vi "ECU Event Page.vi"(8 "error in (no error)":errorcluster, 11 "Node Ptr":T1 format="%.0x") -> (0 "error out":errorcluster)   [LabVIEW 2011, in "Engine Sim System Explorer.lvlib"]
uses:
  Engine Sim System Explorer.lvlib
  <vilib>/NI Veristand/Custom Device API/Custom Device Item Ref.ctl
  Shared/Engine Simulation Global.vi
  <vilib>/NI Veristand/Custom Device API/Get Item Property (Boolean).vi
  <vilib>/NI Veristand/Custom Device API/Get Item Property (Double).vi
  <vilib>/NI Veristand/Custom Device API/Set Item Property (Boolean).vi
  <vilib>/NI Veristand/Custom Device API/Set Item Property (Double).vi
  <vilib>/NI Veristand/Custom Device API/Custom Device API.lvlib
  Engine Simulation Shared.lvlib
panel:
  in  "ParentRate":bool
  in  "FPGA Event Loop Rate (Hz)":dbl format="%#_p"
  in  "SHDocVw.IWebBrowser2":refnum<k7>(container)
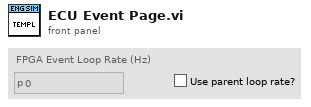
[diagram p1: front panel]
types:
  T1 = typedef "Custom Device API.lvlib/Custom Device Item Ref.ctl" = u64
  T2 = enum8{"Enabled", "Disabled", "Disabled and Grayed Out"}
  T3 = typedef "Custom Device API.lvlib/Custom Device Commands.ctl" = enum16{"Default", "Item renamed", "Shutdown", "Dynamic button pressed"}
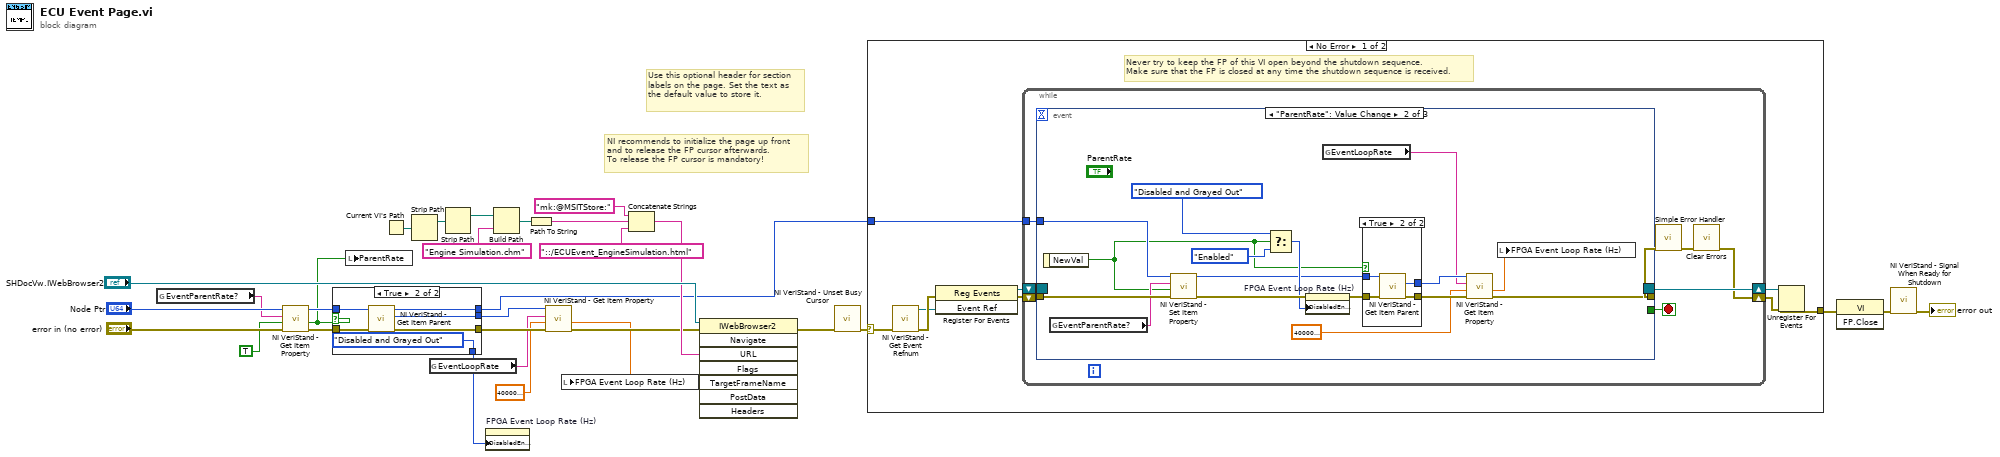
[diagram p0: block diagram]
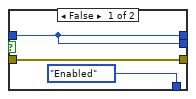
[diagram p2: hidden frame]
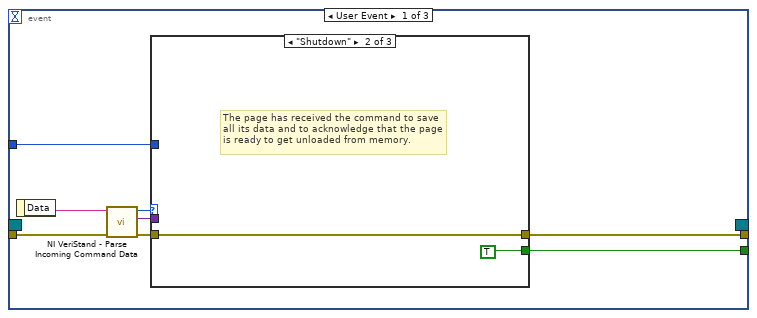
[diagram p3: hidden frame]
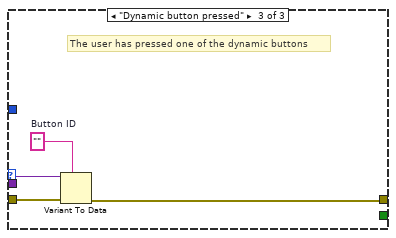
[diagram p5: hidden frame]
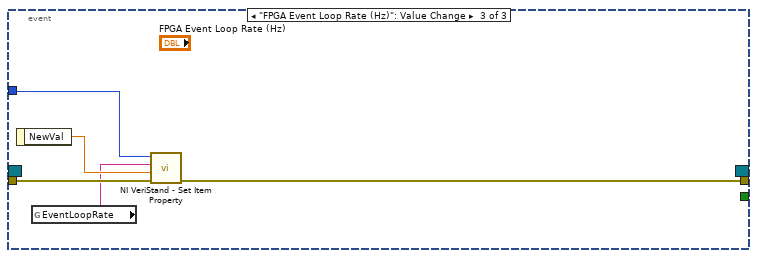
[diagram p7: hidden frame]
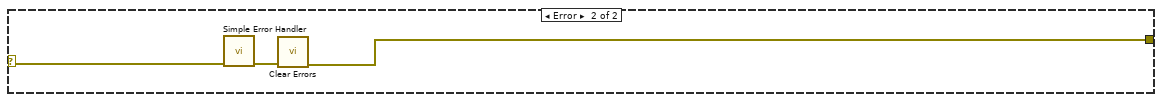
[diagram p8: hidden frame]
diagram:
  # "Use this optional header for section labels on the page. Set the text as the default value to store it."
  # "NI recommends to initialize the page up front\nand to release the FP cursor afterwards.\nTo release the FP cursor is mandatory!"
  n1 = global read "Engine Simulation Global.vi" "EventParentRate?"() -> (w13:string)
  n2 = call-poly <vilib>:"NI VeriStand - Get Item Property.vi"("error in (no error)"="error in (no error)", "Default Value"=TRUE, "Property Name"=w13, "Item Ref in"="Node Ptr") -> ("error out"=w10:errorcluster, "Value"=w9:bool, "Item Ref out"=w11:T1)  [unwired: 4 in, 1 out]
  n3 = case shown="True" w9 {
    tunnel: w11 -> [w32 w39]
    tunnel: w10 -> [w33 w38]
    tunnel: [w33 w37] -> w8
    tunnel: [w32 w36] -> w5
    tunnel: [w32 w35] -> w4
    tunnel: [T2."Enabled" ("Disabled") T2."Disabled and Grayed Out" ("Disabled")] -> w1
    frame False {
    }
    frame True {
      n4 = call <vilib>:"NI VeriStand - Get Item Parent.vi"("error in (no error)"=w38, "Item Ref in"=w39) -> ("error out"=w37:errorcluster, "Parent Ref"=w36:T1, "Item Ref out"=w35:T1)  [unwired: 6 in, 1 out]
    }
  }
  n5 = local write "ParentRate"(w9) -> ()
  n6 = Current VI's Path() -> (path=w17:path)
  n7 = Strip Path(path=w17) -> (stripped path=w18:path)  [unwired: 1 out]
  n8 = global read "Engine Simulation Global.vi" "EventLoopRate"() -> (w6:string)
  n9 = Strip Path(path=w18) -> (stripped path=w23:path)  [unwired: 1 out]
  n10 = property on="FPGA Event Loop Rate (Hz)" class="DigNum (strict)"("DisabledEnum"=w1) -> ()  [unwired: 2 in, 2 out]
  n11 = Build Path(base path=w23, name or relative path="Engine Simulation.chm") -> (appended path=w21:path)
  n12 = Path To String(path=w21) -> (string=w20:string)
  n13 = call-poly <vilib>:"NI VeriStand - Get Item Property.vi"("error in (no error)"=w8, "Default Value"=40000000.0, "Property Name"=w6, "Item Ref in"=w5) -> ("error out"=w7:errorcluster, "Value"=w2:dbl)  [unwired: 4 in, 2 out]
  n14 = local write "FPGA Event Loop Rate (Hz)"(w2) -> ()
  n15 = Concatenate Strings("mk:@MSITStore:" ("string"), w20, "::/ECUEvent_EngineSimulation.html" ("name or relative path")) -> (w15:string)
  n16 = invoke class="IWebBrowser2" method="Navigate"(reference="SHDocVw.IWebBrowser2", error in=w7, "URL"=w15) -> (error out=w27:errorcluster)  [unwired: 5 in, 7 out]
  n17 = call <vilib>:"NI VeriStand - Unset Busy Cursor.vi"("error in (no error)"=w27) -> ("error out"=w26:errorcluster)  [unwired: 10 out]
  n18 = case shown="No Error" w26 {
    selector: w26 -> [w40 w101]
    tunnel: [w45 w99] -> w30
    tunnel: w4 -> [w41 _]
    frame No Error {
      # "Never try to keep the FP of this VI open beyond the shutdown sequence.\nMake sure that the FP is closed at any time the shutdown sequence is received."
      n19 = call <vilib>:"NI VeriStand - Get Event Refnum.vi"("error in (no error)"=w40) -> ("error out"=w48:errorcluster, "Event Ref"=w44:refnum<user-event>)  [unwired: 9 out]
      n20 = register-events(error in=w48, w44) -> (reference out=w42:refnum<event-registration>, error out=w43:errorcluster)  [unwired: 1 in]
      n21 = while {
        tunnel: w41 -> [w52]
        shift-right: [w49] -> w46
        shift-left: w43 -> [w55]
        shift-right: [w56] -> w47
        shift-left: w42 -> [w54]
        stop <- w53 stop-if-true
        n22 = event shown="[1] \"ParentRate\": Value Change" {
          selector: w54 -> [_ _ _]
          dyn-events: [_ _ _] -> w56
          timeout: _ -> [_ _ _]
          tunnel: w55 -> [w64 w87 w98]
          tunnel: [w60 _ _] -> w53
          tunnel: [w59 w72 w94] -> w51
          tunnel: w52 -> [w58 w86 w97]
          event User Event {
            n23 = event-data() -> ("Data"=w63:string)  [unwired: 1 out]
            n24 = call <vilib>:"NI VeriStand - Parse Incoming Command Data.vi"("error in (no error)"=w64, "Incoming data"=w63) -> ("error out"=w62:errorcluster, "Outgoing data"=w57:variant, "Action"=w61:T3)  [unwired: 7 out]
            n25 = case shown="\"Shutdown\"" w61 {
              tunnel: w62 -> [w65 w66 w71]
              tunnel: [_ TRUE _] -> w60
              tunnel: [w65 w66 w68] -> w59
              tunnel: w58 -> [_ _ _]
              tunnel: w57 -> [_ _ w70]
              frame "Default", Default {
              }
              frame "Shutdown" {
                # "The page has received the command to save all its data and to acknowledge that the page is ready to get unloaded from memory."
              }
              frame "Dynamic button pressed" {
                w69 = ""  # Button ID
                # "The user has pressed one of the dynamic buttons"
                n26 = Variant To Data(error in=w71, type=w69, Variant=w70) -> (error out=w68:errorcluster)  [unwired: 1 out]
              }
            }
          }
          event "ParentRate": Value Change {
            n27 = event-data() -> ("NewVal"=w79:bool)  [unwired: 1 out]
            n28 = global read "Engine Simulation Global.vi" "EventParentRate?"() -> (w85:string)
            n29 = call-poly <vilib>:"NI VeriStand - Set Item Property.vi"("error in (no error)"=w87, "Value"=w79, "Property Name"=w85, "Item Ref in"=w86) -> ("error out"=w84:errorcluster, "Item Ref out"=w78:T1)  [unwired: 5 in, 1 out]
            n30 = Select(t=T2."Disabled and Grayed Out" ("Disabled"), s=w79, f=T2."Enabled" ("Disabled")) -> (s? t:f=w81:T2)
            n31 = property on="FPGA Event Loop Rate (Hz)" class="DigNum (strict)"(error in=w84, "DisabledEnum"=w81) -> (error out=w80:errorcluster)  [unwired: 1 in, 1 out]
            n32 = global read "Engine Simulation Global.vi" "EventLoopRate"() -> (w74:string)
            n33 = case shown="True" w79 {
              tunnel: w80 -> [w88 w93]
              tunnel: w78 -> [w89 w92]
              tunnel: [w89 w91] -> w76
              tunnel: [w88 w90] -> w77
              frame False {
              }
              frame True {
                n34 = call <vilib>:"NI VeriStand - Get Item Parent.vi"("error in (no error)"=w93, "Item Ref in"=w92) -> ("error out"=w90:errorcluster, "Parent Ref"=w91:T1)  [unwired: 6 in, 2 out]
              }
            }
            n35 = call-poly <vilib>:"NI VeriStand - Get Item Property.vi"("error in (no error)"=w77, "Default Value"=40000000.0, "Property Name"=w74, "Item Ref in"=w76) -> ("error out"=w72:errorcluster, "Value"=w73:dbl)  [unwired: 4 in, 2 out]
            n36 = local write "FPGA Event Loop Rate (Hz)"(w73) -> ()
          }
          event "FPGA Event Loop Rate (Hz)": Value Change {
            n37 = event-data() -> ("NewVal"=w96:dbl)  [unwired: 1 out]
            n38 = global read "Engine Simulation Global.vi" "EventLoopRate"() -> (w95:string)
            n39 = call-poly <vilib>:"NI VeriStand - Set Item Property.vi"("error in (no error)"=w98, "Value"=w96, "Property Name"=w95, "Item Ref in"=w97) -> ("error out"=w94:errorcluster)  [unwired: 5 in, 2 out]
          }
        }
        n40 = call <vilib>:"Simple Error Handler.vi"("error in (no error)"=w51) -> ("error out"=w50:errorcluster)  [unwired: 1 in, 7 out]
        n41 = call <vilib>:"Clear Errors.vi"("error in (no error)"=w50) -> ("error out"=w49:errorcluster)  [unwired: 6 out]
      }
      n42 = Unregister For Events(event registration refnum=w47, error in=w46) -> (error out=w45:errorcluster)
    }
    frame Error {
      n43 = call <vilib>:"Simple Error Handler.vi"("error in (no error)"=w101) -> ("error out"=w100:errorcluster)  [unwired: 1 in, 7 out]
      n44 = call <vilib>:"Clear Errors.vi"("error in (no error)"=w100) -> ("error out"=w99:errorcluster)  [unwired: 6 out]
    }
  }
  n45 = invoke class="VI" method="FP.Close"(error in=w30) -> (error out=w29:errorcluster)  [unwired: 2 in, 2 out]
  n46 = call <vilib>:"NI VeriStand - Signal When Ready for Shutdown.vi"("error in (no error)"=w29) -> ("error out"=→"error out":errorcluster)  [unwired: 10 out]
